vi "example.vi"() -> ()   [LabVIEW 2021]
uses:
  <vilib>/Analysis/6fits.llb/Curve Fitting Criteria.ctl
  <vilib>/Analysis/baseanly.llb/Mean (DBL).vi
  <vilib>/Analysis/NI_AALPro.lvlib
  <vilib>/Analysis/NI_AALBase.lvlib
panel:
  out "MAE Least Square":dbl format="%0.2f"
  out "MAE Theil-Sen":dbl format="%0.2f"
  out "intercept":dbl
  out "slope":dbl
  out "XY Graph":cluster{dbl[], dbl[]}[](graph)
  out "b":dbl format="%.6g"
  out "m":dbl format="%.6g"
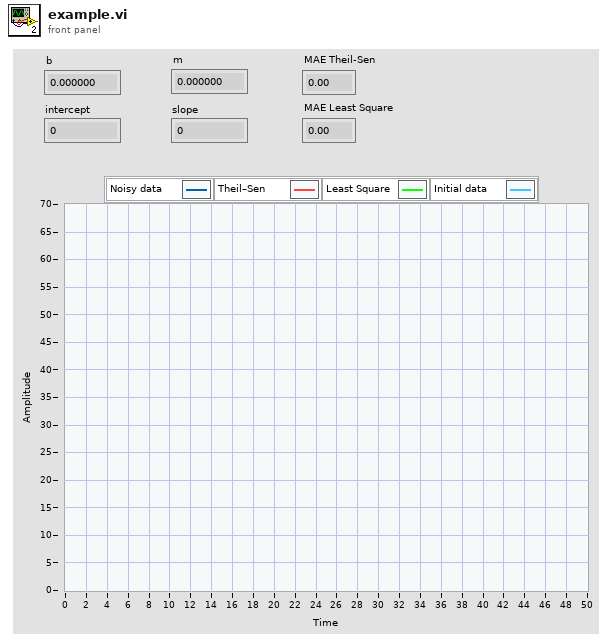
[diagram p1: front panel]
types:
  T1 = typedef "NI_AALPro.lvlib/Curve Fitting Criteria.ctl" = u16
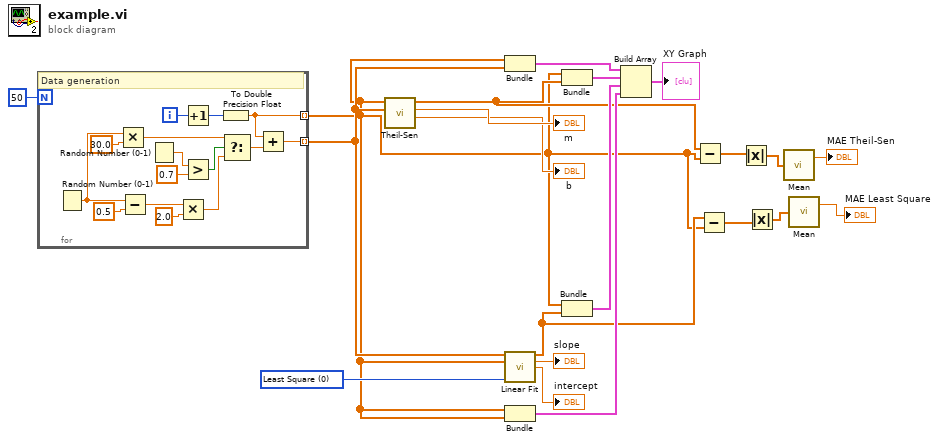
[diagram p0: block diagram]
diagram:
  w16 = T1 0 items=["Least Square", "Least Absolute Residual", "Bisquare"] ("method")
  n1 = for {
    N: 50 -> [_]
    tunnel: [w31] -> w1 mode=indexing
    tunnel: [w34] -> w8 mode=indexing
    i -> [w33]
    # "Data generation"
    n2 = Random Number (0-1)() -> (number: 0 to 1=w24:dbl)
    n3 = Multiply(x=w24, y=30.0 ("t")) -> (x*y=w23:dbl)
    n4 = Subtract(x=w24, y=0.5) -> (x-y=w36:dbl)
    n5 = Random Number (0-1)() -> (number: 0 to 1=w30:dbl)
    n6 = Multiply(x=w36, y=2.0) -> (x*y=w27:dbl)
    n7 = Increment(x=w33) -> (x+1=w32:i32)
    n8 = Greater?(x=w30, y=0.7) -> (0:w26:bool)
    n9 = To Double Precision Float(number=w32) -> (double precision float=w31:dbl)
    n10 = Select(t=w23, s=w26, f=w27) -> (s? t:f=w22:dbl)
    n11 = Add(x=w31, y=w22) -> (x+y=w34:dbl)
  }
  n12 = call "Theil-Sen.vi"("input_Y"=w8, "input_X"=w1) -> ("b"=→"b":dbl, "m"=→"m":dbl, "output_Y"=w10:dbl[])  [unwired: 4 in, 1 out]
  n13 = Bundle(w1, w8) -> (w20:cluster{dbl[], dbl[]})  [unwired: 1 in]
  n14 = call <vilib>:"Linear Fit.vi"("Y"=w8, "X"=w1, "method"=w16) -> ("Best Linear Fit"=w9:dbl[], "slope"=→"slope":dbl, "intercept"=→"intercept":dbl)  [unwired: 8 in, 2 out]
  n15 = Bundle(w1, w1) -> (w17:cluster{dbl[], dbl[]})  [unwired: 1 in]
  n16 = Bundle(w1, "output_Y"=w10) -> (w19:cluster{dbl[], "output_Y":dbl[]})  [unwired: 1 in]
  n17 = Bundle(w1, "Best Linear Fit"=w9) -> (w15:cluster{dbl[], "Best Linear Fit":dbl[]})  [unwired: 1 in]
  n18 = Build Array(w20, w19, w15, w17) -> (→"XY Graph":cluster{dbl[], "Best Linear Fit":dbl[]}[])
  n19 = Subtract(x=w10, y=w1) -> (x-y=w7:dbl[])
  n20 = Subtract(x=w9, y=w1) -> (x-y=w6:dbl[])
  n21 = Absolute Value(x=w7) -> (abs(x)=w5:dbl[])
  n22 = Absolute Value(x=w6) -> (abs(x)=w4:dbl[])
  n23 = call-poly <vilib>:"Mean.vi"("X"=w5) -> ("mean"=→"MAE Theil-Sen":dbl)  [unwired: 1 out]
  n24 = call-poly <vilib>:"Mean.vi"("X"=w4) -> ("mean"=→"MAE Least Square":dbl)  [unwired: 1 out]
